vi "Project 2 (Main).vi"() -> ()   [LabVIEW 2018]
doc: "Mian VI for realizing control of the LED light stuick using LabVIEW in EE 200 Project 2."
uses:
  controls/Enum Defining FSM State.ctl
  controls/Cluster for displaying  ABR switch states.ctl
  controls/Cluster for displaying  LED outputs.ctl
  controls/Enum Defining myDAQ Actions.ctl
  controls/Enum Defining FGV Action.ctl
panel:
  out "LED Outputs":T1
  out "User Inputs":T2
  in  "Stop Button":bool
  out "Present State":T3
  out "Clock Cycle":i32
  # "LED Light Stick Controller"
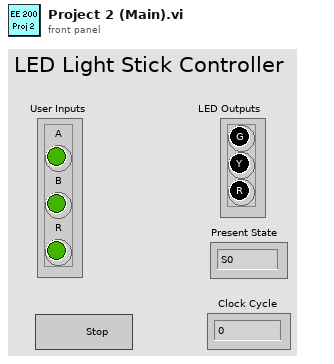
[diagram p1: front panel]
types:
  T1 = typedef "Cluster for displaying  LED outputs.ctl" = cluster{"G":bool, "Y":bool, "R":bool}
  T2 = typedef "Cluster for displaying  ABR switch states.ctl" = cluster{"A":bool, "B":bool, "R":bool}
  T3 = typedef "Enum Defining FSM State.ctl" = enum16{"S0", "S1", "S2", "S3"}
  T4 = typedef "Enum Defining myDAQ Actions.ctl" = enum16{"Initilialize", "Read Buttons", "Set LED Lights", "Release"}
  T5 = typedef "Enum Defining FGV Action.ctl" = enum16{"Set", "Get"}
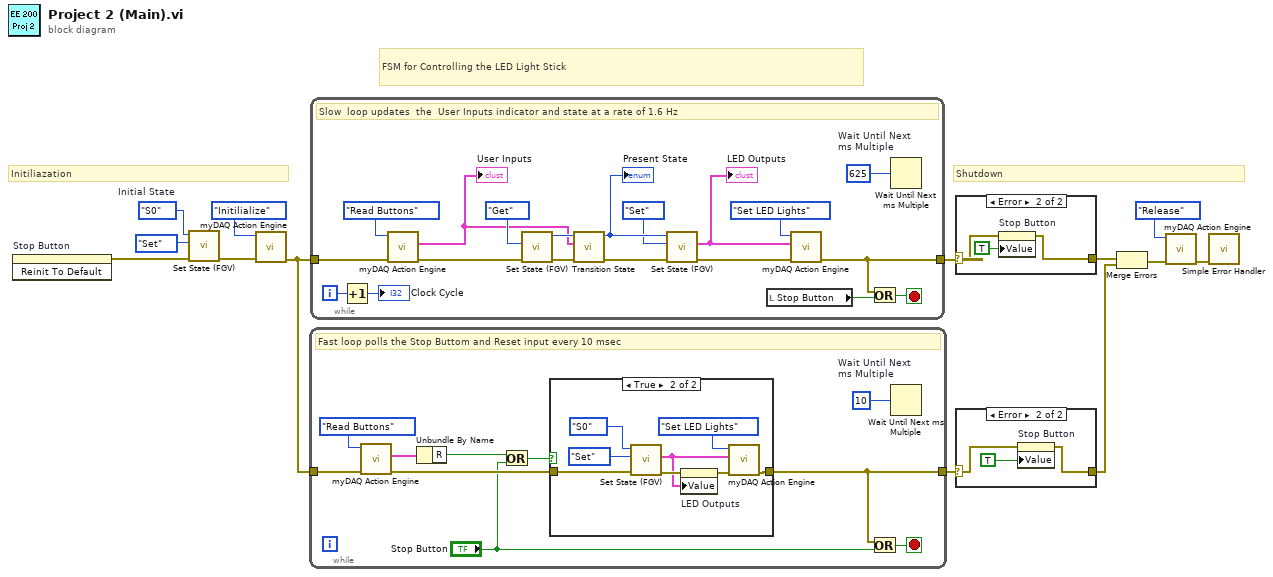
[diagram p0: block diagram]
diagram:
  w11 = Enum_Defining_FSM_State."S0"  # Initial State
  # "Shutdown"
  # "Initiliazation"
  # "FSM for Controlling the LED Light Stick"
  n1 = invoke on="Stop Button" class="Bool (strict)" method="Reinit To Default"() -> (error out=w2:errorcluster)  [unwired: 3 in, 2 out]
  n2 = call "Set State (FGV).vi"("Error In"=w2, "Action"=Enum_Defining_FGV_Action."Set", "State Input"=w11) -> ("Error Out"=w12:errorcluster)  [unwired: 6 in, 2 out]
  n3 = call "myDAQ Action Engine.vi"("Error In"=w12, "Enum Defining myDAQ Action"=Enum_Defining_myDAQ_Actions."Initilialize") -> ("Error Out"=w10:errorcluster)  [unwired: 8 in, 1 out]
  n4 = while {
    tunnel: w10 -> [w22]
    tunnel: [w19] -> w8
    stop <- w20 stop-if-true
    # "Fast loop polls the Stop Buttom and Reset input every 10 msec"
    n5 = call "myDAQ Action Engine.vi"("Error In"=w22, "Enum Defining myDAQ Action"=Enum_Defining_myDAQ_Actions."Read Buttons" ("Enum Defining DIO Action")) -> ("Error Out"=w21:errorcluster, "Inputs"=w15:T2)  [unwired: 8 in]
    n6 = Unbundle By Name(w15) -> ("R"=w14:bool)
    n7 = Or(x=w14, y="Stop Button") -> (x .or. y?=w17:bool)
    n8 = case shown="True" w17 {
      tunnel: w21 -> [w24 w31]
      tunnel: [w24 w29] -> w19
      frame False {
      }
      frame True {
        n9 = call "Set State (FGV).vi"("Error In"=w31, "Action"=Enum_Defining_FGV_Action."Set", "State Input"=Enum_Defining_FSM_State."S0" ("Input State")) -> ("Error Out"=w26:errorcluster, "Controller Output"=w25:T1)  [unwired: 6 in, 1 out]
        n10 = property on="LED Outputs" class="Clust (strict)"("Value"=w25) -> ()  [unwired: 2 in, 2 out]
        n11 = call "myDAQ Action Engine.vi"("Error In"=w26, "Controller Output"=w25, "Enum Defining myDAQ Action"=Enum_Defining_myDAQ_Actions."Set LED Lights" ("Enum Defining DIO Action")) -> ("Error Out"=w29:errorcluster)  [unwired: 7 in, 1 out]
      }
    }
    n12 = Or(x=w19, y="Stop Button") -> (x .or. y?=w20:bool)
    n13 = Wait Until Next ms Multiple "Wait Until Next \nms Multiple"(millisecond multiple=u32 10 ("millisecond\nmultiple")) -> ()  [unwired: 1 out]
  }
  n14 = while {
    tunnel: w10 -> [w48]
    tunnel: [w43] -> w9
    i -> [w50]
    stop <- w42 stop-if-true
    # "Slow  loop updates  the  User Inputs indicator and state at a rate of 1.6 Hz"
    n15 = Increment(x=w50) -> (x+1=→"Clock Cycle":i32)
    n16 = call "myDAQ Action Engine.vi"("Error In"=w48, "Enum Defining myDAQ Action"=Enum_Defining_myDAQ_Actions."Read Buttons" ("Enum Defining DIO Action")) -> ("Error Out"=w41:errorcluster, "Inputs"=w33:T2)  [unwired: 8 in]
    "User Inputs" <- w33
    n17 = call "Set State (FGV).vi"("Error In"=w41, "Action"=Enum_Defining_FGV_Action."Get") -> ("Error Out"=w40:errorcluster, "State Output"=w39:T3)  [unwired: 7 in, 1 out]
    n18 = call "Transition State.vi"("Error In"=w40, "Inputs"=w33, "Present  State"=w39) -> ("Error Out"=w46:errorcluster, "Next State"=w45:T3)  [unwired: 7 in]
    "Present State" <- w45
    n19 = call "Set State (FGV).vi"("Error In"=w46, "Action"=Enum_Defining_FGV_Action."Set", "State Input"=w45) -> ("Error Out"=w44:errorcluster, "Controller Output"=w32:T1)  [unwired: 6 in, 1 out]
    "LED Outputs" <- w32
    n20 = local read "Stop Button"() -> (w37:bool)
    n21 = call "myDAQ Action Engine.vi"("Error In"=w44, "Controller Output"=w32, "Enum Defining myDAQ Action"=Enum_Defining_myDAQ_Actions."Set LED Lights" ("Enum Defining DIO Action")) -> ("Error Out"=w43:errorcluster)  [unwired: 7 in, 1 out]
    n22 = Or(x=w43, y=w37) -> (x .or. y?=w42:bool)
    n23 = Wait Until Next ms Multiple "Wait Until Next \nms Multiple"(millisecond multiple=u32 625 ("millisecond\nmultiple")) -> ()  [unwired: 1 out]
  }
  n24 = case shown="Error" w9 {
    selector: w9 -> [w51 w53]
    tunnel: [w51 w52] -> w7
    frame No Error {
    }
    frame Error {
      n25 = property on="Stop Button" class="Bool (strict)"(error in=w53, "Value"=TRUE ("Stop Button")) -> (error out=w52:errorcluster)  [unwired: 1 in, 1 out]
    }
  }
  n26 = case shown="Error" w8 {
    selector: w8 -> [w55 w57]
    tunnel: [w55 w58] -> w6
    frame No Error {
    }
    frame Error {
      n27 = property on="Stop Button" class="Bool (strict)"(error in=w57, "Value"=TRUE ("Stop Button")) -> (error out=w58:errorcluster)  [unwired: 1 in, 1 out]
    }
  }
  n28 = Merge Errors(w7, w6) -> (w5:errorcluster)
  n29 = call "myDAQ Action Engine.vi"("Error In"=w5, "Enum Defining myDAQ Action"=Enum_Defining_myDAQ_Actions."Release") -> ("Error Out"=w4:errorcluster)  [unwired: 8 in, 1 out]
  n30 = call <vilib>:"Simple Error Handler.vi"("error in (no error)"=w4) -> ()  [unwired: 4 in, 5 out]
